vi "Histeresis.vi"() -> ()   [LabVIEW 2020]
panel:
  out "LED":bool
  out "Escalar":dbl
  in  "Min":dbl
  in  "Máx":dbl
  out "Arreglo de datos":dbl[](array[numeric])
  # "Diego Jáuregui Ontiveros\nCarlos Uriel Casas Casas\nAlejandro López González"
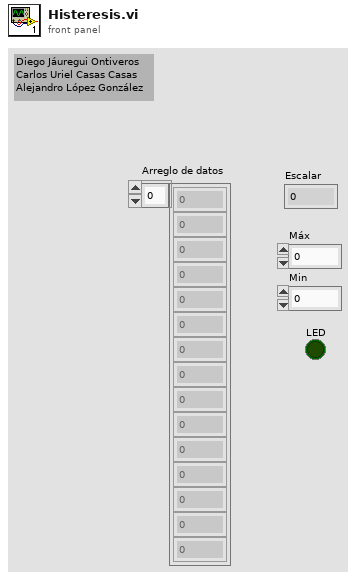
[diagram p1: front panel]
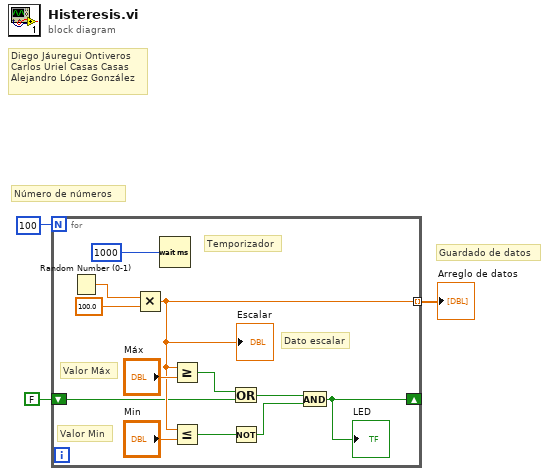
[diagram p0: block diagram]
diagram:
  # "Guardado de datos"
  # "Número de números"
  # "Diego Jáuregui Ontiveros\nCarlos Uriel Casas Casas\nAlejandro López González"
  n1 = for {
    N: 100 -> [_]
    tunnel: [w11] -> w3 mode=indexing
    shift-right: [w5] -> _
    shift-left: FALSE -> [w9]
    # "Valor Min"
    # "Valor Máx"
    # "Dato escalar"
    # "Temporizador"
    n2 = Random Number (0-1)() -> (number: 0 to 1=w14:dbl)
    n3 = Multiply(x=w14, y=100.0 ("x*y")) -> (x*y=w11:dbl)
    "Escalar" <- w11
    n4 = Wait (ms)(milliseconds to wait=u32 1000) -> ()  [unwired: 1 out]
    n5 = Greater Or Equal?(x=w11, y="Máx") -> (x >= y?=w4:bool)
    n6 = Less Or Equal?(x=w11, y="Min") -> (x <= y?=w8:bool)
    n7 = Or(x=w4, y=w9) -> (x .or. y?=w6:bool)
    n8 = Not(x=w8) -> (.not. x?=w7:bool)
    n9 = And(x=w6, y=w7) -> (x .and. y?=w5:bool)
    "LED" <- w5
  }
  "Arreglo de datos" <- w3
